vi "Insert Front Panel.vi"(8 "error in (no error)":errorcluster, 9 "Insertion Request Time":timestamp, 10 "Protected Subpanel":T1, 11 "Login View in":refnum<class "Login View.lvclass">) -> (0 "error out":errorcluster, 3 "Login View out":refnum<class "Login View.lvclass">)   [LabVIEW 2017, in "Login View.lvlib" / "Login View.lvclass"]
doc: "<License>\nCopyright © 2017 Composed Systems, LLC | All rights reserved\nwww.composed.io\n\nAuthor: Ethan Stern <ethan.stern@composed.io>\n\nThis software is provided \"AS IS\" WITHOUT WARRANTIES, either express or implied, AND IS FOR EDUCATIONAL PURPOSES ONLY.\n</License>"
uses:
  Login View.lvclass
  <vilib>/gpm_packages/@cs/mva-viewable/Source/IViewable/ProtectedSubpanel/Protected Subpanel Reference.ctl
  <vilib>/gpm_packages/@cs/mva-viewable/Source/IViewable/ProtectedSubpanel/ProtectedSubpanel.lvclass
  Login View.lvclass/Login View.ctl
  <vilib>/gpm_packages/@cs/mva-viewable/Source/IViewable/IViewable/IViewable.lvclass
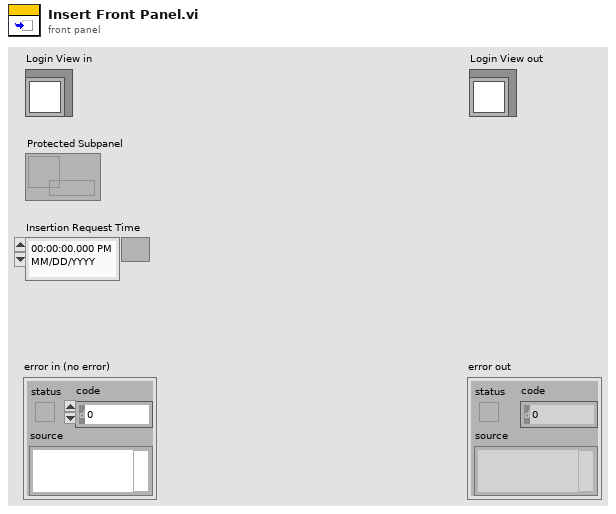
[diagram p1: front panel]
types:
  T1 = typedef "IViewable.lvlib/ProtectedSubpanel.lvclass/Protected Subpanel Reference.ctl" = refnum<data-value>
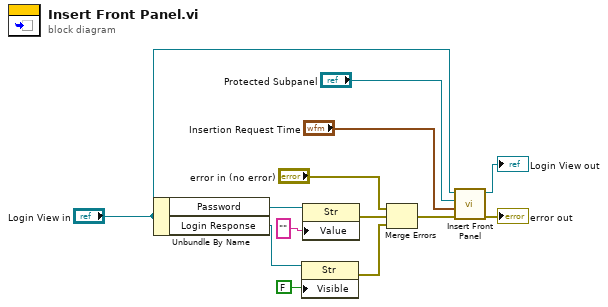
[diagram p0: block diagram]
diagram:
  n1 = Unbundle By Name("Login View in") -> ("Password"=w8:refnum<vi>, "Login Response"=w6:refnum<vi>)
  n2 = property on="Property Node" class="Str"(reference=w6, "Visible"=FALSE) -> (error out=w4:errorcluster)  [unwired: 1 in, 1 out]
  n3 = property on="Property Node" class="Str"(reference=w8, "Value"="") -> (error out=w3:errorcluster)  [unwired: 1 in, 1 out]
  n4 = Merge Errors("error in (no error)", w3, w4) -> (w1:errorcluster)
  n5 = call-parent "Insert Front Panel.vi"("error in (no error)"=w1, "Insertion Request Time"="Insertion Request Time", "Protected Subpanel"="Protected Subpanel", "IViewable in"="Login View in") -> ("error out"=→"error out":errorcluster, "IViewable out"=→"Login View out":refnum<class "Login View.lvclass">)  [unwired: 6 in]
